vi "Create.vi"(8 "error in (no error)":errorcluster, 9 "Loader Name":string, 10 "pid":u32, 11 "Plugin Manager in":refnum<class "CIFPluginLoader.lvclass">) -> (0 "error out":errorcluster, 3 "Plugin Manager out":refnum<class "CIFPluginLoader.lvclass">)   [LabVIEW 2021, in "CIFPluginLoader.lvclass"]
uses:
  CIFPluginLoader.lvclass
  <vilib>/CIF Foundation/CIF Core/CIFUtilities/CIFLogs/Typedef/Message Type.ctl
  typedef/Loaded Plugin Map.ctl
  <vilib>/CIF Foundation/CIF Core/CIFPluginManager/gRPC/CIF_Manager_client/RPC Messages/cif_management_common_LoaderInfoFull.ctl
  <vilib>/CIF Foundation/CIF Core/CIFPluginManager/gRPC/CIF_Manager_client/RPC Messages/cif_management_common_LoaderType.ctl
  CIFPluginLoader.lvclass/CIFPluginLoader.ctl
  <vilib>/CIF Foundation/CIF Core/CIFUtilities/CIFConfigurationFile/CIF Configuration File.lvlib
  <vilib>/CIF Foundation/CIF Core/CIFUtilities/CIFLogs/CIFLogs.lvlib
  <vilib>/CIF Foundation/CIF Core/CIFPluginManager/gRPC/CIF_Manager_Client_Wrapper/CIFManagerClientWrapper.lvlib
  <vilib>/CIF Foundation/CIF Core/CIFPluginManager/gRPC/CIF_Manager_client/CIF_Manager_client.lvlib
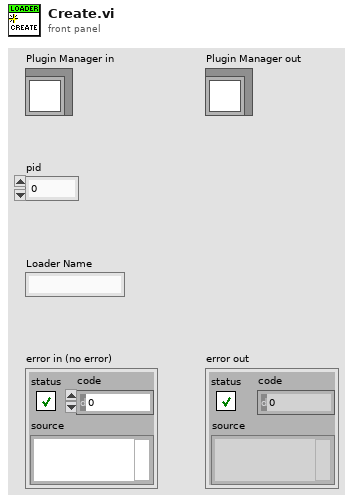
[diagram p1: front panel]
types:
  T1 = typedef "CIF_Manager_client.lvlib/cif_management_common_LoaderType.ctl" = enum32{"LOADERTYPE_UNKNOWN", "LOADERTYPE_LABVIEW"}
  T2 = typedef "CIF_Manager_client.lvlib/cif_management_common_LoaderInfoFull.ctl" = cluster{"loader_type":T1, "loader_name":string, "grpc_port":i32, "pid":u32}
  T3 = typedef "CIFPluginLoader.lvclass/Loaded Plugin Map.ctl" = map{string, refnum<vi>}
  T4 = typedef "CIFLogs.lvlib/Message Type.ctl" = enum16{"Error", "Information", "Print Terminal", "Configuration"}
  T5 = typedef "grpc-lvsupport-release.lvlib/grpcId.ctl" = u64
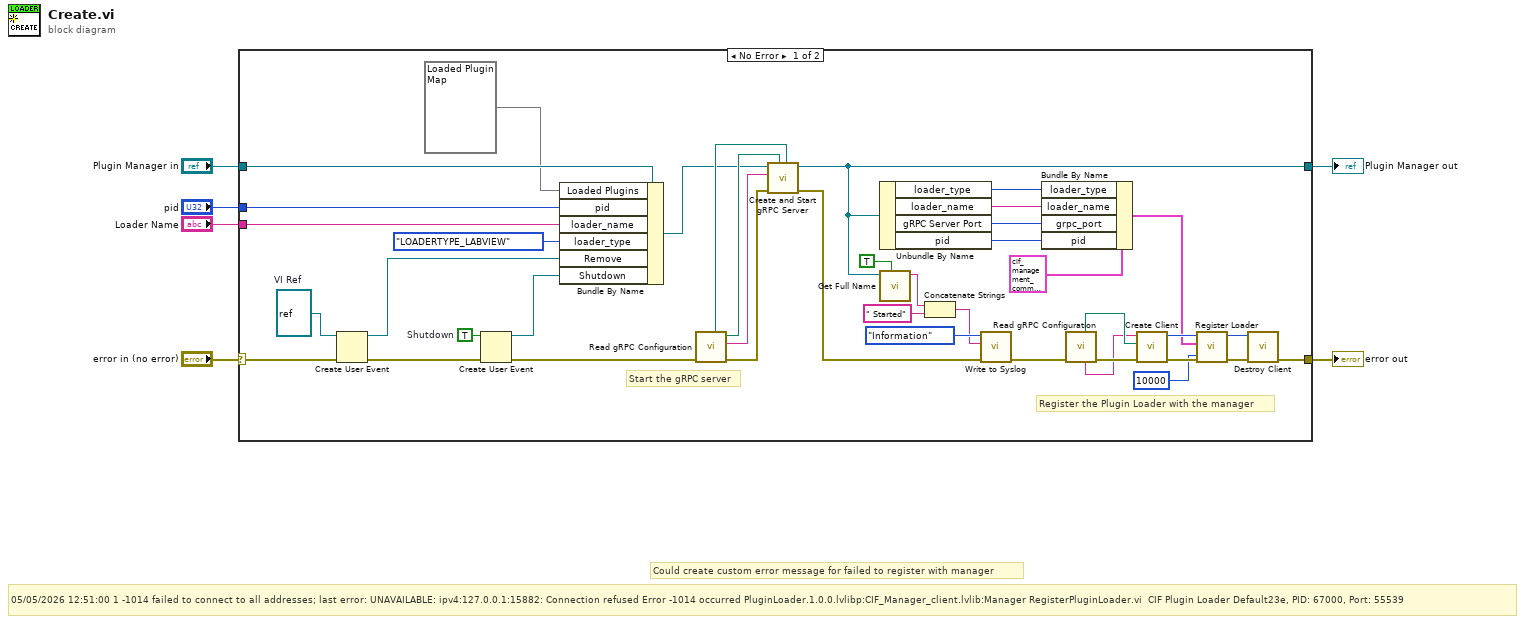
[diagram p0: block diagram]
diagram:
  # "05/05/2026 12:51:00\t1\t-1014\tfailed to connect to all addresses; last error: UNAVAILABLE: ipv4:127.0.0.1:15882: Connection refused\tError -1014 occurred PluginLoader.1.0.0.lvlibp:CIF_Manager_client.lvlib:Manager RegisterPluginLoader.vi \tCIF Plugin Loader Default23e, PID: 67000, Port: 55539"
  # "Could create custom error message for failed to register with manager"
  n1 = case shown="No Error" "error in (no error)" {
    selector: "error in (no error)" -> [w11 w48]
    tunnel: [w17 w48] -> w5
    tunnel: [w28 w47] -> w3
    tunnel: "Plugin Manager in" -> [w39 w47]
    tunnel: "pid" -> [w30 _]
    tunnel: "Loader Name" -> [w36 _]
    frame No Error {
      w9 = refnum<vi> refnum  # VI Ref
      w42 = TRUE  # Shutdown
      # "Register the Plugin Loader with the manager"
      # "Start the gRPC server"
      n2 = Create User Event(user event datatype=w9, error in=w11) -> (user event=w7:refnum<user-event>, error out=w10:errorcluster)
      n3 = Create User Event(user event datatype=w42, error in=w10) -> (user event=w8:refnum<user-event>, error out=w41:errorcluster)
      n4 = Bundle By Name(cluster=w39, "Loaded Plugins"=T3 {}, "pid"=w30, "loader_name"=w36, "loader_type"=cif_management_common_LoaderType."LOADERTYPE_LABVIEW", "Remove"=w7, "Shutdown"=w8) -> (w37:refnum<class "CIFPluginLoader.lvclass">)
      n5 = call <vilib>:"Read gRPC Configuration.vi"("error in"=w41) -> ("error out"=w46:errorcluster, "Plugin Server Address"=w31:string, "Server Certificate File (.crt)"=w44:path, "Server Key File (.key)"=w45:path)  [unwired: 5 in, 2 out]
      n6 = call "Create and Start gRPC Server.vi"("Server Key File (.key)"=w45, "Server Certificate File (.crt)"=w44, "error in (no error)"=w46, "Server Address"=w31, "CIFLauncher in"=w37) -> ("error out"=w40:errorcluster, "CIFLauncher out"=w28:refnum<class "CIFPluginLoader.lvclass">)  [unwired: 5 in]
      n7 = Unbundle By Name(w28) -> ("loader_type"=w15:T1, "loader_name"=w14:string, "gRPC Server Port"=w33:i32, "pid"=w32:u32)
      n8 = call "Get Full Name.vi"("Include Extra Info"=TRUE, "CIFPluginLoader in"=w28) -> ("Name"=w29:string)  [unwired: 9 in]
      n9 = Concatenate Strings(w29, " Started" ("message")) -> (w27:string)
      n10 = call <vilib>:"Write to Syslog.vi"("error in (no error)"=w40, "message"=w27, "CIF Message Type"=Message_Type."Information") -> ("error out"=w34:errorcluster)  [unwired: 8 in]
      n11 = Bundle By Name(cluster=T2 {"loader_type"=enum."LOADERTYPE_UNKNOWN", "loader_name"="", "grpc_port"=0, "pid"=0} ("Loader Info"), "loader_type"=w15, "loader_name"=w14, "grpc_port"=w33, "pid"=w32) -> (w25:T2)
      n12 = call <vilib>:"Read gRPC Configuration.vi"("error in"=w34) -> ("error out"=w20:errorcluster, "Local Manager Address"=w18:string, "Server Key File (.key)"=w19:path)  [unwired: 5 in, 3 out]
      n13 = call <vilib>:"Create Client.vi"("error in"=w20, "Server Certificate File (.crt)"=w19, "address"=w18) -> ("error out"=w24:errorcluster, "gRPC ID Out"=w26:T5)  [unwired: 7 in]
      n14 = call <vilib>:"Register Loader.vi"("timeout (ms)"=10000, "error in"=w24, "Loader Info"=w25, "gRPC ID in"=w26) -> ("error out"=w23:errorcluster, "gRPC ID out"=w22:T5)  [unwired: 6 in]
      n15 = call <vilib>:"Destroy Client.vi"("error in"=w23, "gRPC ID"=w22) -> ("error out"=w17:errorcluster)  [unwired: 9 in]
    }
    frame Error {
    }
  }
  "error out" <- w5
  "Plugin Manager out" <- w3
